vi "UpdateSetup.vi"(8 "error in (no error)":errorcluster, 10 "data":u16, 11 "Caculator in":refnum<class "Caculator.lvclass">) -> (0 "error out":errorcluster, 3 "Caculator out":refnum<class "Caculator.lvclass">)   [LabVIEW 2017, in "Caculator.lvclass"]
uses:
  Caculator.lvclass
  Caculator.lvclass/Caculator.ctl
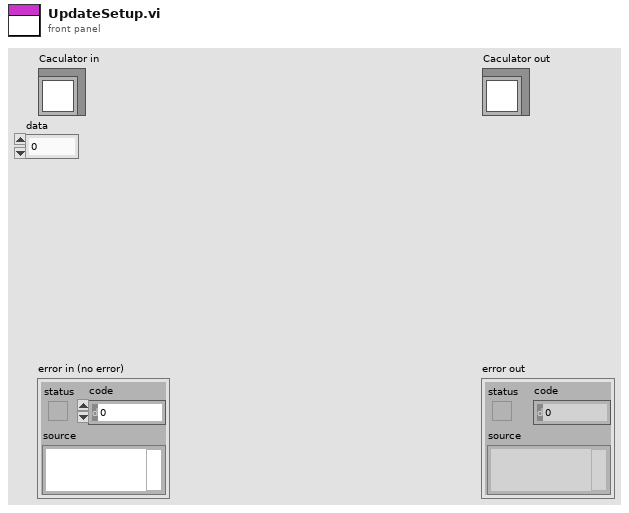
[diagram p1: front panel]
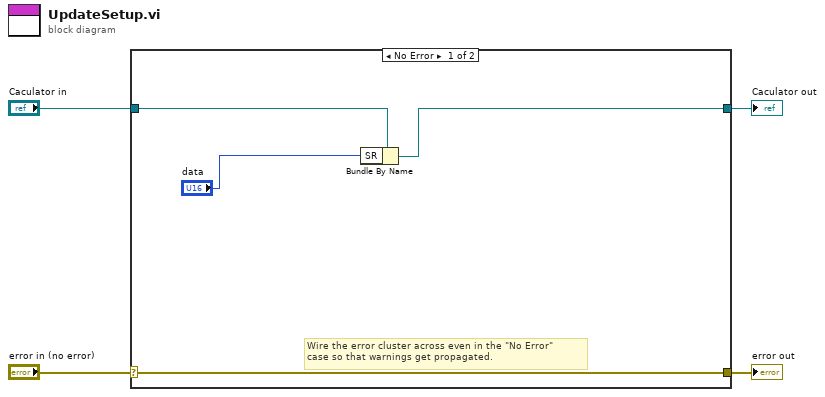
[diagram p0: block diagram]
diagram:
  n1 = case shown="No Error" "error in (no error)" {
    selector: "error in (no error)" -> [w8 w10]
    tunnel: [w8 w10] -> w3
    tunnel: [w6 w9] -> w1
    tunnel: "Caculator in" -> [w7 w9]
    frame No Error {
      # "Wire the error cluster across even in the \"No Error\"\ncase so that warnings get propagated."
      n2 = Bundle By Name(cluster=w7, "SR"="data") -> (w6:refnum<class "Caculator.lvclass">)
    }
    frame Error {
    }
  }
  "error out" <- w3
  "Caculator out" <- w1
